vi "Format Class Info Column.vi"(8 "error in (no error)":errorcluster {"code" format="Error %.0f"}, 9 "Column":T1, 10 "Class_Library":T2, 11 "VIDoc Printer - Confluence In":refnum<class "VIDoc Printer - Confluence.lvclass">) -> (0 "error out":errorcluster {"code" format="Error %.0f"}, 1 "Header":string, 2 "Cell Text":string, 3 "VIDoc Printer - Confluence Out":refnum<class "VIDoc Printer - Confluence.lvclass">, 4 "Viable Value?":bool, 5 "Pixel Width":i16=275)   [LabVIEW 2023, in "VIDoc Printer - Confluence.lvlib" / "VIDoc Printer - Confluence.lvclass"]
uses:
  VIDoc Printer - Confluence.lvclass
  Parsing/TypeDefs/Base Class Info Cluster.ctl
  <vilib>/picture/picture.llb/imagedata.ctl
  Settings/Confluence Printer Settings/Class Info Column.ctl
  <userlib>/_PetranWay/LabVIEW Confluence API/Source/Confluence/HTML/Add Link to Text/Add URL to Text.vi
  VIDoc Printer - Confluence.lvclass/VIDoc Printer - Confluence.ctl
  Printer/VIDoc Printer.lvclass
  <userlib>/_PetranWay/LabVIEW Confluence API/Source/PetranWay_Confluence API.lvlib
  Parsing/VIDoc Parsing.lvlib
  Settings/Confluence Printer Settings/VIDoc Settings - Confluence.lvclass
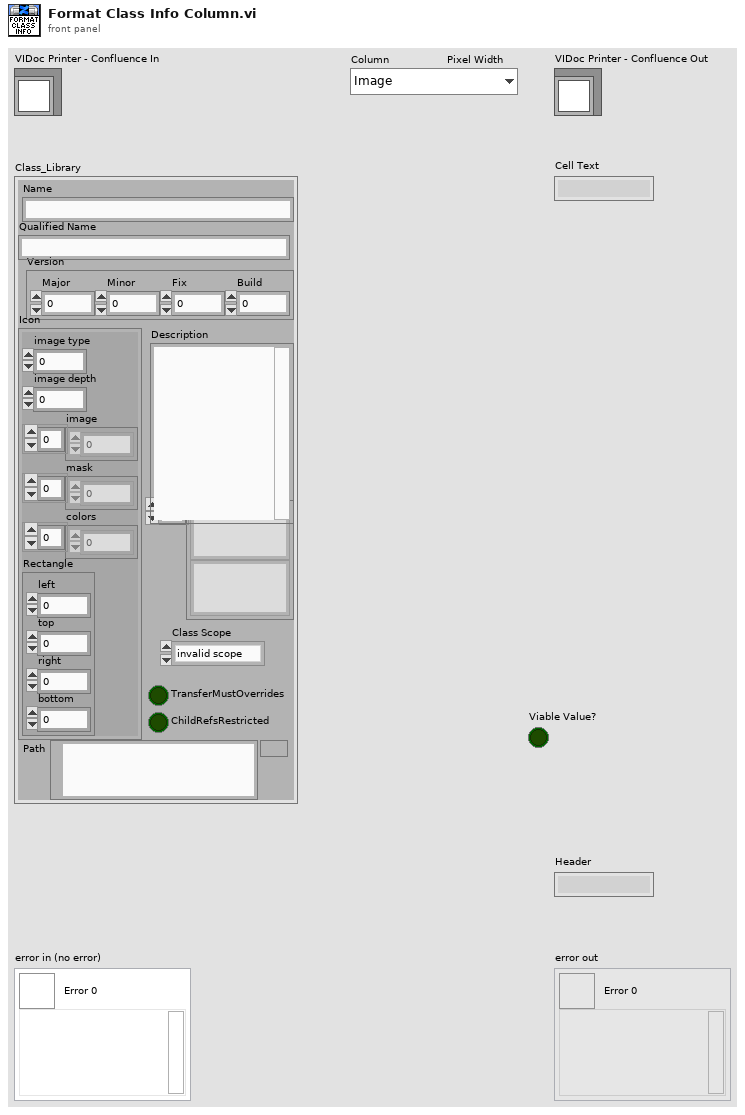
[diagram p1: front panel]
types:
  T1 = typedef "VIDoc Printer - Confluence.lvlib/VIDoc Settings - Confluence.lvclass/Class Info Column.ctl" = enum16{"Image", "Name", "Description", "Version", "Last Change", "Author", "Commit Hash", "Branch", "Qualified Name", "TransferMustOverrides", "ChildRefsRestricted"}
  T2 = typedef "VIDoc Parsing.lvlib/Base Class Info Cluster.ctl" = cluster{"Name":string, "Icon":T3, "Version":cluster{"Major":u16, "Minor":u16, "Fix":u16, "Build":u16}, "Description":string, "Friends":string[], "ChildRefsRestricted":bool, "TransferMustOverrides":bool, "Path":path, "Qualified Name":string, "Class Scope":enum32{"invalid scope", "public", "private", "protected", "community"}}
  T3 = typedef "imagedata.ctl" = cluster{"image type":i32, "image depth":i32, "image":u8[], "mask":u8[], "colors":u32[], "Rectangle":cluster{"left":i16, "top":i16, "right":i16, "bottom":i16}}
  T4 = cluster{"Major":u16, "Minor":u16, "Fix":u16, "Build":u16}
  T5 = cluster{"Timestamp":timestamp, "Commit Hash":string, "Author Name":string, "Branch":string, "Commit Hash URL":string}
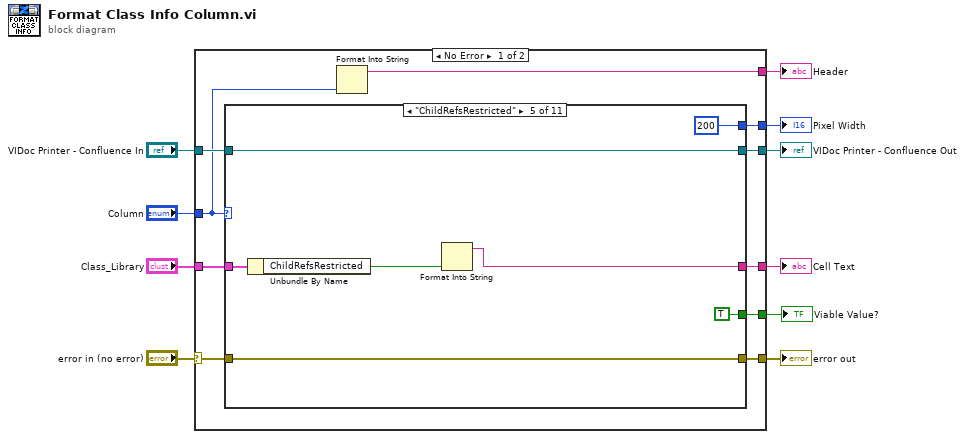
[diagram p0: block diagram]
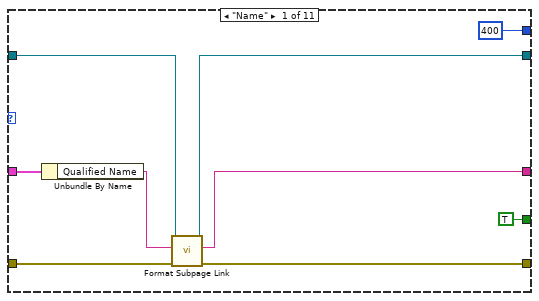
[diagram p2: hidden frame]
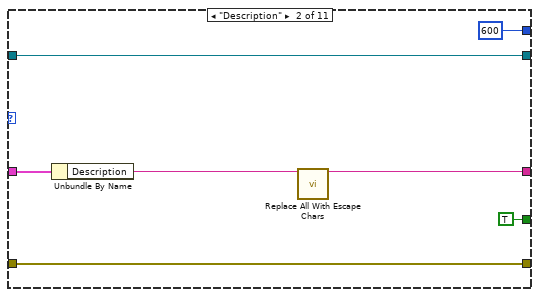
[diagram p3: hidden frame]
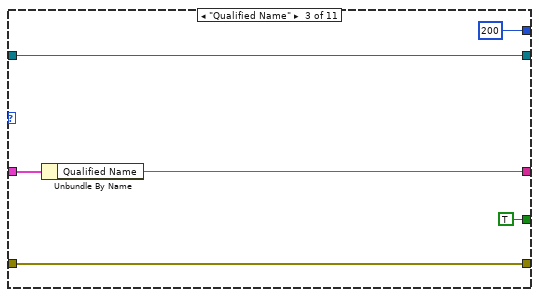
[diagram p4: hidden frame]
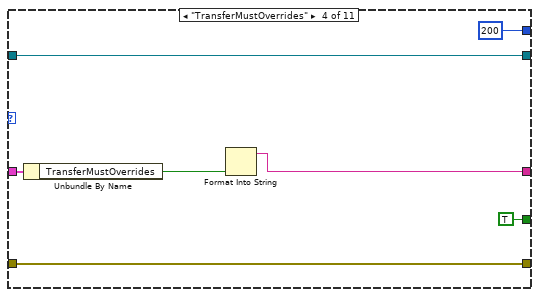
[diagram p5: hidden frame]
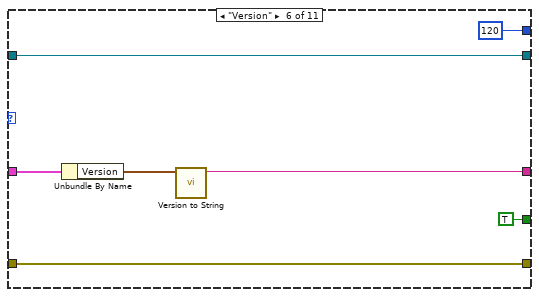
[diagram p6: hidden frame]
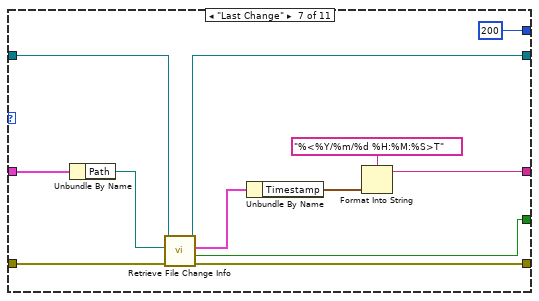
[diagram p7: hidden frame]
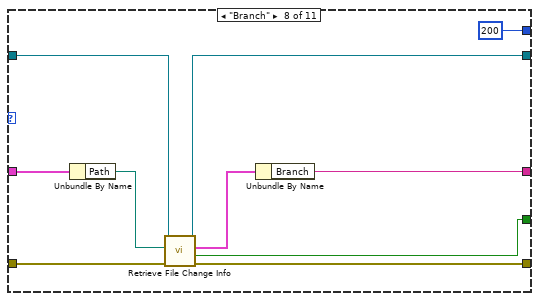
[diagram p8: hidden frame]
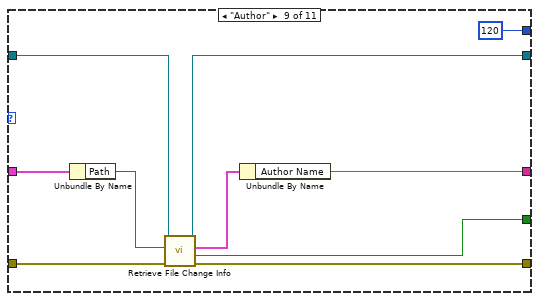
[diagram p9: hidden frame]
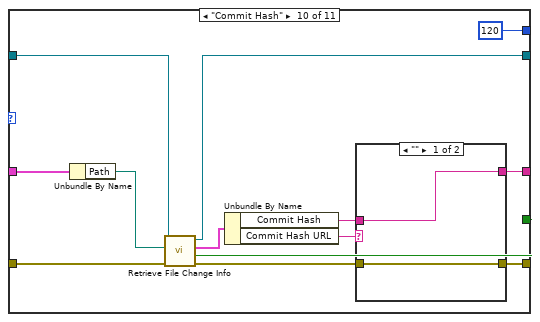
[diagram p10: hidden frame]
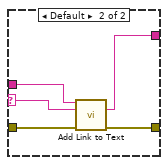
[diagram p11: hidden frame]
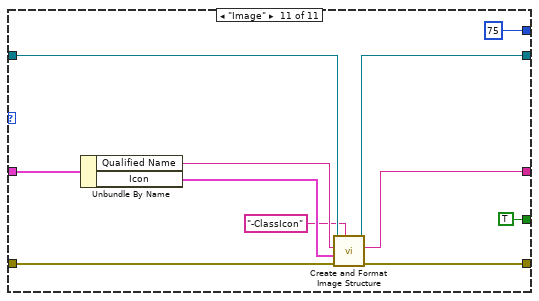
[diagram p12: hidden frame]
diagram:
  n1 = case shown="No Error" "error in (no error)" {
    selector: "error in (no error)" -> [w17 w128]
    tunnel: [w18 w128] -> w9
    tunnel: [w20 w127] -> w7
    tunnel: "VIDoc Printer - Confluence In" -> [w19 w127]
    tunnel: "Column" -> [w16 _]
    tunnel: [w15 _] -> w5
    tunnel: [w14 _] -> w4
    tunnel: "Class_Library" -> [w13 _]
    tunnel: [w12 _] -> w2
    tunnel: [w11 _] -> w1
    frame No Error {
      n2 = case shown="\"ChildRefsRestricted\"" w16 {
        tunnel: [w25 w33 w39 w46 w53 w60 w67 w79 w89 w101 w121] -> w20
        tunnel: w19 -> [w24 w33 w39 w46 w53 w60 w66 w78 w88 w103 w122]
        tunnel: [w27 w34 w40 w47 w54 w61 w69 w81 w91 w96 w117] -> w18
        tunnel: w17 -> [w26 w34 w40 w47 w54 w61 w70 w82 w92 w105 w123]
        tunnel: [i16 400 ("Pixel Width") i16 600 ("Pixel Width") i16 200 ("Pixel Width") i16 200 ("Pixel Width") i16 200 ("Pixel Width") i16 120 ("Pixel Width") i16 200 ("Pixel Width") i16 200 ("Pixel Width") i16 120 ("Pixel Width") i16 120 ("Pixel Width") i16 75 ("Pixel Width")] -> w14
        tunnel: w13 -> [w28 w35 w41 w48 w55 w62 w74 w84 w94 w107 w124]
        tunnel: [w22 w30 w38 w43 w50 w58 w65 w77 w87 w99 w116] -> w12
        tunnel: [TRUE ("File Change Info Available?") TRUE ("File Change Info Available?") TRUE ("File Change Info Available?") TRUE ("File Change Info Available?") TRUE ("File Change Info Available?") TRUE ("File Change Info Available?") w64 w76 w86 w102 TRUE ("File Change Info Available?")] -> w11
        frame "Name" {
          n3 = Unbundle By Name(w28) -> ("Qualified Name"=w23:string)
          n4 = call "Format Subpage Link.vi"("error in (no error)"=w26, "Qualified Name"=w23, "VIDoc Printer - Confluence In"=w24) -> ("error out"=w27:errorcluster, "Linked HTML"=w22:string, "VIDoc Printer - Confluence Out"=w25:refnum<class "VIDoc Printer - Confluence.lvclass">)  [unwired: 6 in]
        }
        frame "Description" {
          n5 = Unbundle By Name(w35) -> ("Description"=w32:string)
          n6 = call <userlib>:"Replace All With Escape Chars.vi"("Raw String"=w32) -> ("With Substitued Escape Characters"=w30:string)  [unwired: 13 in, 1 out]
        }
        frame "Qualified Name" {
          n7 = Unbundle By Name(w41) -> ("Qualified Name"=w38:string)
        }
        frame "TransferMustOverrides" {
          n8 = Unbundle By Name(w48) -> ("TransferMustOverrides"=w44:bool)
          n9 = Format Into String(w44) -> (resulting string=w43:string)  [unwired: 3 in, 1 out]
        }
        frame "ChildRefsRestricted" {
          n10 = Unbundle By Name(w55) -> ("ChildRefsRestricted"=w51:bool)
          n11 = Format Into String(w51) -> (resulting string=w50:string)  [unwired: 3 in, 1 out]
        }
        frame "Version" {
          n12 = Unbundle By Name(w62) -> ("Version"=w59:T4)
          n13 = call "Version to String.vi"("Version"=w59) -> ("String"=w58:string)  [unwired: 10 in]
        }
        frame "Last Change" {
          n14 = Unbundle By Name(w74) -> ("Path"=w68:path)
          n15 = call "Retrieve File Change Info.vi"("error in (no error)"=w70, "Absolute File Path"=w68, "VIDoc Printer - Confluence In"=w66) -> ("error out"=w69:errorcluster, "File Change Info Available?"=w64:bool, "File Change Info"=w73:T5, "VIDoc Printer - Confluence Out"=w67:refnum<class "VIDoc Printer - Confluence.lvclass">)  [unwired: 5 in]
          n16 = Unbundle By Name(w73) -> ("Timestamp"=w72:timestamp)
          n17 = Format Into String(format string="%<%Y/%m/%d %H:%M:%S>T", w72) -> (resulting string=w65:string)  [unwired: 2 in, 1 out]
        }
        frame "Branch" {
          n18 = Unbundle By Name(w84) -> ("Path"=w80:path)
          n19 = call "Retrieve File Change Info.vi"("error in (no error)"=w82, "Absolute File Path"=w80, "VIDoc Printer - Confluence In"=w78) -> ("error out"=w81:errorcluster, "File Change Info Available?"=w76:bool, "File Change Info"=w83:T5, "VIDoc Printer - Confluence Out"=w79:refnum<class "VIDoc Printer - Confluence.lvclass">)  [unwired: 5 in]
          n20 = Unbundle By Name(w83) -> ("Branch"=w77:string)
        }
        frame "Author" {
          n21 = Unbundle By Name(w94) -> ("Path"=w90:path)
          n22 = call "Retrieve File Change Info.vi"("error in (no error)"=w92, "Absolute File Path"=w90, "VIDoc Printer - Confluence In"=w88) -> ("error out"=w91:errorcluster, "File Change Info Available?"=w86:bool, "File Change Info"=w93:T5, "VIDoc Printer - Confluence Out"=w89:refnum<class "VIDoc Printer - Confluence.lvclass">)  [unwired: 5 in]
          n23 = Unbundle By Name(w93) -> ("Author Name"=w87:string)
        }
        frame "Commit Hash" {
          n24 = Unbundle By Name(w107) -> ("Path"=w104:path)
          n25 = call "Retrieve File Change Info.vi"("error in (no error)"=w105, "Absolute File Path"=w104, "VIDoc Printer - Confluence In"=w103) -> ("error out"=w97:errorcluster, "File Change Info Available?"=w102:bool, "File Change Info"=w106:T5, "VIDoc Printer - Confluence Out"=w101:refnum<class "VIDoc Printer - Confluence.lvclass">)  [unwired: 5 in]
          n26 = Unbundle By Name(w106) -> ("Commit Hash"=w100:string, "Commit Hash URL"=w98:string)
          n27 = case shown="\"\"" w98 {
            selector: w98 -> [_ w113]
            tunnel: w100 -> [w110 w115]
            tunnel: [w110 w114] -> w99
            tunnel: w97 -> [w109 w112]
            tunnel: [w109 w111] -> w96
            frame "" {
            }
            frame Default {
              n28 = call-poly <userlib>:"Add Link to Text.vi"("Text"=w115, "URL"=w113, "error in (no error)"=w112) -> ("HTML Text String"=w114:string, "error out"=w111:errorcluster)  [unwired: 10 in, 1 out]
            }
          }
        }
        frame "Image" {
          n29 = Unbundle By Name(w124) -> ("Qualified Name"=w120:string, "Icon"=w119:T3)
          n30 = call "Create and Format Image Structure.vi"("Name Addition"="-ClassIcon" ("string"), "Error in"=w123, "Image Data"=w119, "Name"=w120, "VIDoc Printer - Confluence In"=w122) -> ("Error out"=w117:errorcluster, "Image Structure Text"=w116:string, "VIDoc Printer - Confluence Out"=w121:refnum<class "VIDoc Printer - Confluence.lvclass">)  [unwired: 3 in, 1 out]
        }
      }
      n31 = Format Into String(w16) -> (resulting string=w15:string)  [unwired: 3 in, 1 out]
    }
    frame Error {
    }
  }
  "error out" <- w9
  "VIDoc Printer - Confluence Out" <- w7
  "Pixel Width" <- w4
  "Cell Text" <- w2
  "Header" <- w5
  "Viable Value?" <- w1
